vi "URAPI_Micro_Delay_num.vi"(0 "Time In":u32=1, 3 "URAPI Script":T1={"Script"="", "Whiles"=[], "Ifs"=[], "Supress Err"=TRUE, "Errors"=""}) -> (5 "URAPI Script out":T1={"Script"="", "Whiles"=[], "Ifs"=[], "Supress Err"=TRUE, "Errors"=""})   [LabVIEW 2012]
doc: "Causes the script to wait the specified number of seconds before continuing to execute."
uses:
  <userlib>/BotSpeak/VIs/Direct/URAPI_Control.ctl
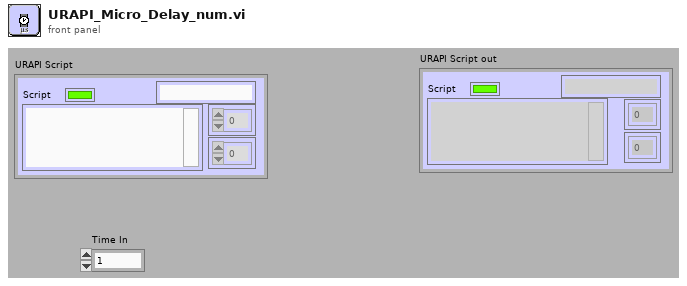
[diagram p1: front panel]
types:
  T1 = typedef "URAPI_Control.ctl" = cluster{"Script":string, "Whiles":u8[], "Ifs":u8[], "Supress Err":bool, "Errors":string}
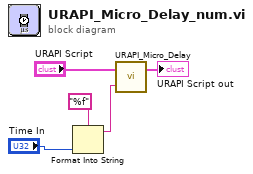
[diagram p0: block diagram]
diagram:
  n1 = Format Into String(format string="%f" ("string"), "Time In") -> (resulting string=w2:string)  [unwired: 2 in, 1 out]
  n2 = call <userlib>:"URAPI_Micro_Delay.vi"("Variable In"=w2, "URAPI Script"="URAPI Script") -> ("URAPI Script out"=→"URAPI Script out":T1)  [unwired: 3 in]
